vi "escribeEnTablaUnValor.vi"(8 "element":dbl, 9 "fila":i32, 10 "col":i32=2, 11 "tabla in":string[][](array[string])) -> (3 "tabla out":string[][](array[string]))   [LabVIEW 2019, in "Prueba.lvclass"]
uses:
  Prueba.lvclass
panel:
  out "x = y?":bool
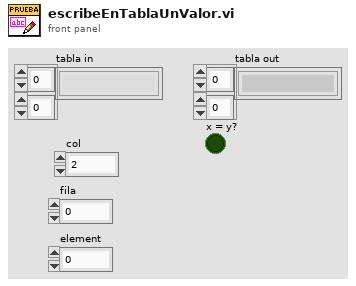
[diagram p1: front panel]
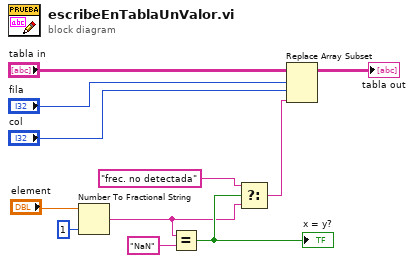
[diagram p0: block diagram]
diagram:
  n1 = Number To Fractional String(number="element", precision (6)=i16 1) -> (F-format string=w2:string)  [unwired: 2 in]
  n2 = Equal?(x=w2, y="NaN") -> (x = y?=w4:bool)
  "x = y?" <- w4
  n3 = Select(t="frec. no detectada" ("y"), s=w4, f=w2) -> (s? t:f=w1:string)
  n4 = Replace Array Subset(array="tabla in", new element=w1, index (row)="fila", index (col)="col") -> (→"tabla out":string[][])
